vi "Parametric Linear Piecewise Function.vi"(9 "Points":dbl[][](array[numeric]), 11 "Parametric\nValue":dbl) -> (2 "Y Position":dbl, 3 "X Position":dbl)   [LabVIEW 2017]
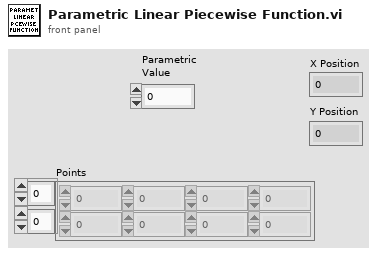
[diagram p1: front panel]
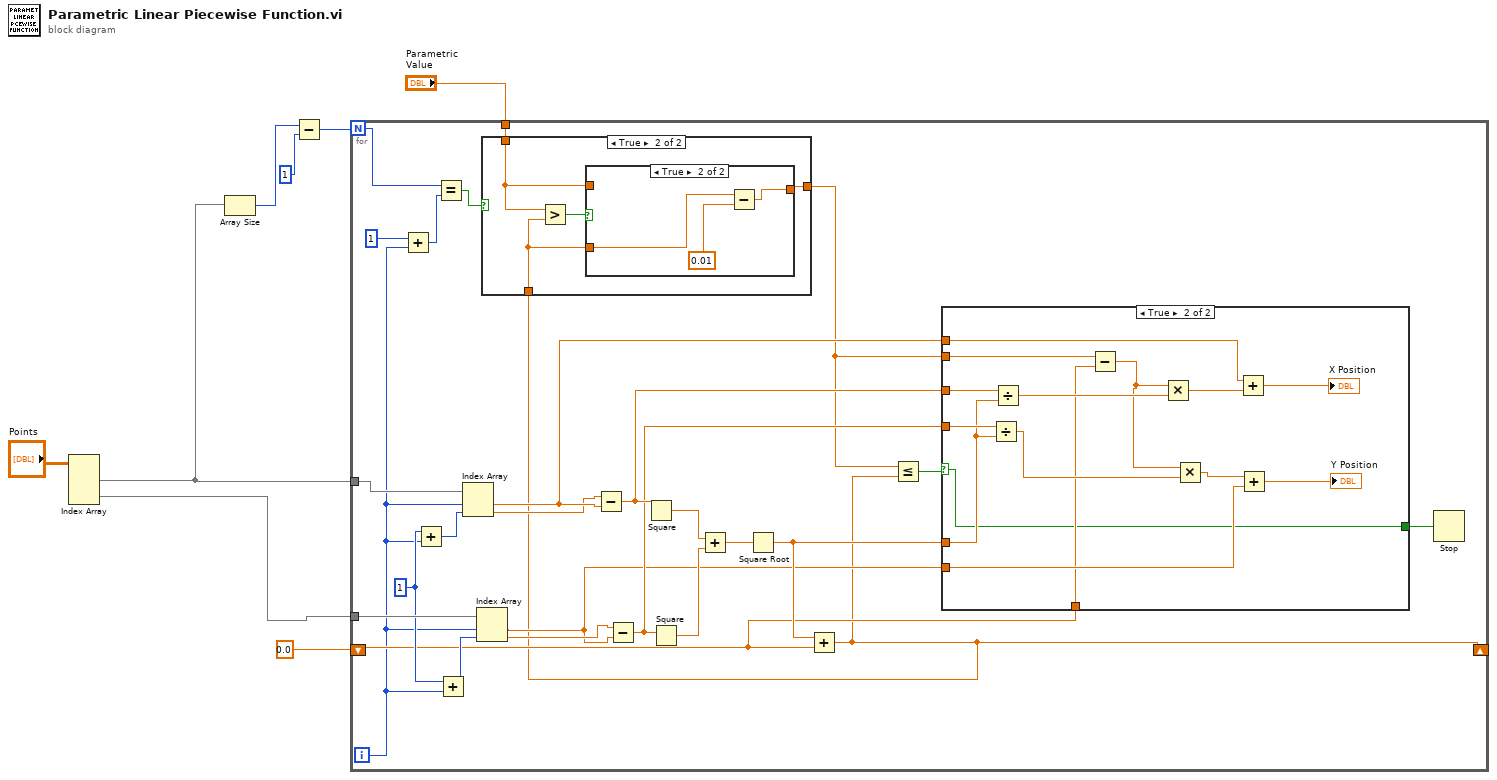
[diagram p0: block diagram]
diagram:
  n1 = Index Array(array="Points") -> (element #1=w5:dbl[], element #2=w6:dbl[])  [unwired: 4 in]
  n2 = Array Size(array=w5) -> (size(s)=w3:i32)
  n3 = Subtract(x=w3, y=1) -> (x-y=w4:i32)
  n4 = for {
    N: w4 -> [w13]
    tunnel: w5 -> [w34]
    tunnel: w6 -> [w32]
    shift-right: [w11] -> _
    shift-left: 0.0 -> [w18]
    tunnel: "Parametric\nValue" -> [w10]
    i -> [w15]
    w30 = 1
    n5 = Add(x=1 ("y"), y=w15) -> (x+y=w14:i32)
    n6 = Add(x=w30, y=w15) -> (x+y=w33:i32)
    n7 = Equal?(x=w13, y=w14) -> (x = y?=w12:bool)
    n8 = Add(x=w30, y=w15) -> (x+y=w31:i32)
    n9 = Index Array(array=w34, index #1=w15, index #2=w33) -> (element #1=w22:dbl, element #2=w21:dbl)
    n10 = Index Array(array=w32, index #1=w15, index #2=w31) -> (element #1=w19:dbl, element #2=w20:dbl)
    n11 = Subtract(x=w21, y=w22) -> (x-y=w25:dbl)
    n12 = Subtract(x=w20, y=w19) -> (x-y=w24:dbl)
    n13 = Square(x=w25) -> (x^2=w29:dbl)
    n14 = Square(x=w24) -> (x^2=w28:dbl)
    n15 = Add(x=w29, y=w28) -> (x+y=w27:dbl)
    n16 = Square Root(x=w27) -> (sqrt(x)=w23:dbl)
    n17 = Add(x=w23, y=w18) -> (x+y=w11:dbl)
    n18 = case shown="True" w12 {
      tunnel: w11 -> [_ w37]
      tunnel: w10 -> [w35 w38]
      tunnel: [w35 w36] -> w9
      frame False {
      }
      frame True {
        n19 = Greater?(x=w38, y=w37) -> (0:w39:bool)
        n20 = case shown="True" w39 {
          tunnel: w38 -> [w40 _]
          tunnel: w37 -> [_ w43]
          tunnel: [w40 w41] -> w36
          frame False {
          }
          frame True {
            n21 = Subtract(x=w43, y=0.01) -> (x-y=w41:dbl)
          }
        }
      }
    }
    n22 = Less Or Equal?(x=w9, y=w11) -> (x <= y?=w26:bool)
    n23 = case shown="True" w26 {
      selector: w26 -> [w44 w45]
      tunnel: w25 -> [_ w59]
      tunnel: w24 -> [_ w58]
      tunnel: w23 -> [_ w57]
      tunnel: w9 -> [_ w56]
      tunnel: w22 -> [_ w50]
      tunnel: w19 -> [_ w49]
      tunnel: w18 -> [_ w46]
      tunnel: [w44 w45] -> w17
      frame False {
      }
      frame True {
        n24 = Divide(x=w58, y=w57) -> (x/y=w54:dbl)
        n25 = Divide(x=w59, y=w57) -> (x/y=w55:dbl)
        n26 = Subtract(x=w56, y=w46) -> (x-y=w53:dbl)
        n27 = Multiply(x=w53, y=w55) -> (x*y=w52:dbl)
        n28 = Multiply(x=w53, y=w54) -> (x*y=w51:dbl)
        n29 = Add(x=w50, y=w52) -> (x+y=→"X Position":dbl)
        n30 = Add(x=w51, y=w49) -> (x+y=→"Y Position":dbl)
      }
    }
    n31 = Stop(stop? (T)=w17) -> ()
  }
